vi "PQgetvalue.vi"(8 "error in (no error)":errorcluster, 9 "column_number":i32, 10 "row_number":i32, 11 "res":u32) -> (0 "error out":errorcluster, 3 "field_value":string)   [LabVIEW 2019, in "libpqlv.lvlib"]
doc: "Returns a single field value of one row of a PGresult. Row and column numbers start at 0. The caller should not free the result directly. It will be freed when the associated PGresult handle is passed to PQclear."
uses:
  libpqlv.lvlib
  libpq.dll
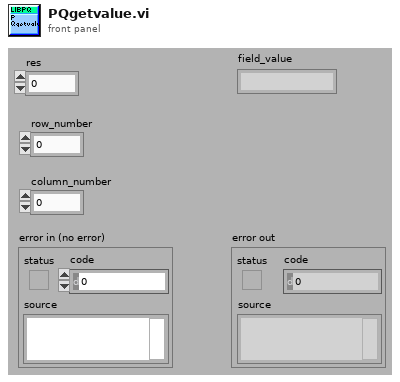
[diagram p1: front panel]
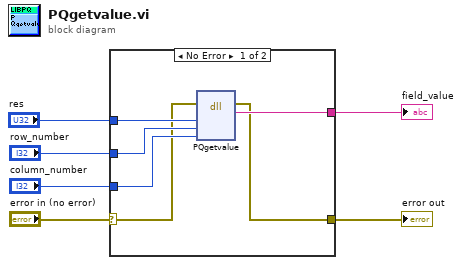
[diagram p0: block diagram]
diagram:
  n1 = case shown="No Error" "error in (no error)" {
    selector: "error in (no error)" -> [w7 w13]
    tunnel: [w8 w13] -> w5
    tunnel: [w12 _] -> w4
    tunnel: "row_number" -> [w11 _]
    tunnel: "column_number" -> [w10 _]
    tunnel: "res" -> [w9 _]
    frame No Error {
      n2 = dll-call lib="libpq.*" fn="PQgetvalue"(error in=w7, "res"=w9, "row_number"=w11, "column_number"=w10) -> (error out=w8:errorcluster, "field_value"=w12:string)  [unwired: 5 in, 1 out]
    }
    frame Error {
    }
  }
  "field_value" <- w4
  "error out" <- w5
